vi "Anritsu VNA Read Start and Stop Frequencies.vi"(6 "Channel":i8=1 min=1 max=99 step=1, 7 "Anritsu VNA":T1, 8 "error in (no error)":errorcluster, 11 "VISA Resource Name":refnum<visa-resource-name>) -> (0 "error out":errorcluster, 2 "Start/Stop Freqs, MHz":cluster{"Fstart":dbl, "Fstop":dbl}, 3 "dup VISA Resource Name":refnum<visa-resource-name>)   [LabVIEW 2011]
doc: "This VI for the HP8753B Network Analyzers reads the stimulus values. Except when performing log sweeps and freq list sweeps, this VI uses the start and stop values and the number of points to calcuate the stimulus values."
uses:
  TypeDefs/Anritsu VNA Instrument Info.ctl
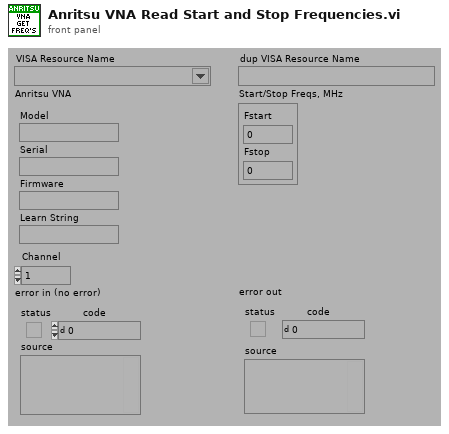
[diagram p1: front panel]
types:
  T1 = typedef "Anritsu VNA Instrument Info.ctl" = cluster{"Model":string, "Serial":string, "Firmware":string, "Learn String":string}
  T2 = typedef "Anritsu VNA Sweep Type.ctl" = enum32{"Linear Sweep", "Frequency Sweep", "Power Sweep", "CW Time Sweep", "Discrete Fill", "Time Domain", "Logarithmic Sweep", "Segmented Sweep (Frequency)", "Segmented Sweep (Index)", "MFGC"}
  T3 = typedef "Anritsu VNA Model.ctl" = enum16{"Not Supported", "37XXXX", "MS20XXX", "MS462XX", "MS464XX"}
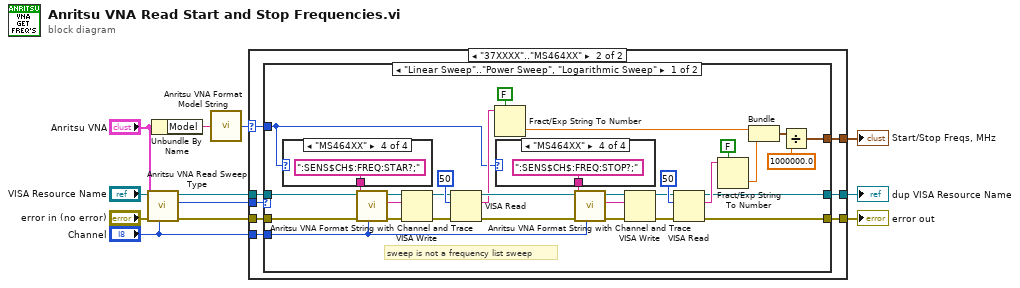
[diagram p0: block diagram]
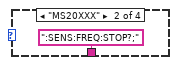
[diagram p4: hidden frame]
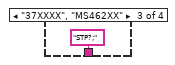
[diagram p5: hidden frame]
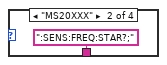
[diagram p7: hidden frame]
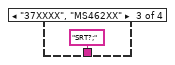
[diagram p8: hidden frame]
diagram:
  n1 = call "Anritsu VNA Read Sweep Type.vi"("Channel"="Channel", "Anritsu VNA"="Anritsu VNA", "error in (no error)"="error in (no error)", "VISA Resource Name"="VISA Resource Name") -> ("error out"=w7:errorcluster, "Sweep Type"=w10:T2, "dup VISA Resource Name"=w8:refnum<visa-resource-name>)  [unwired: 5 out]
  n2 = Unbundle By Name("Anritsu VNA") -> ("Model"=w3:string)
  n3 = call "Anritsu VNA Format Model String.vi"("Model"=w3) -> ("Model"=w2:T3)
  n4 = case shown="\"37XXXX\"..\"MS464XX\"" w2 {
    selector: w2 -> [_ w16]
    tunnel: [w13 w22] -> w12
    tunnel: w10 -> [_ w21]
    tunnel: w8 -> [w14 w20]
    tunnel: w7 -> [w13 w19]
    tunnel: [_ w18] -> w6
    tunnel: [w14 w17] -> w5
    tunnel: "Channel" -> [_ w15]
    frame "Not Supported" {
    }
    frame "37XXXX".."MS464XX" {
      n5 = case shown="\"Linear Sweep\"..\"Power Sweep\", \"Logarithmic Sweep\"" w21 {
        tunnel: w20 -> [w36 w57]
        tunnel: w19 -> [w35 w56]
        tunnel: [w43 w56] -> w22
        tunnel: [w28 _] -> w18
        tunnel: [w30 w57] -> w17
        tunnel: w16 -> [w29 _]
        tunnel: w15 -> [w23 _]
        frame "Linear Sweep".."Power Sweep", "Logarithmic Sweep" {
          # "sweep is not a frequency list sweep"
          n6 = case shown="\"MS464XX\"" w29 {
            tunnel: [_ ":SENS:FREQ:STAR?;" "SRT?;" ":SENS$CH$:FREQ:STAR?;"] -> w27
            frame "Not Supported" {
            }
            frame "MS20XXX" {
            }
            frame "37XXXX", "MS462XX" {
            }
            frame "MS464XX" {
            }
          }
          n7 = call "Anritsu VNA Format String with Channel and Trace.vi"("Channel"=w23, "String"=w27) -> ("String Out"=w26:string)  [unwired: 1 in, 6 out]
          n8 = VISA Write(VISA resource name=w36, write buffer=w26, error in (no error)=w35) -> (VISA resource name out=w39:refnum<visa-resource-name>, error out=w49:errorcluster)  [unwired: 1 out]
          n9 = VISA Read(VISA resource name=w39, byte count=u32 50, error in (no error)=w49) -> (VISA resource name out=w47:refnum<visa-resource-name>, read buffer=w45:string, error out=w46:errorcluster)  [unwired: 1 out]
          n10 = Fract/Exp String To Number(use system decimal point (T)=FALSE, string=w45) -> (number=w33:dbl)  [unwired: 3 out]
          n11 = case shown="\"MS464XX\"" w29 {
            tunnel: [_ ":SENS:FREQ:STOP?;" "STP?;" ":SENS$CH$:FREQ:STOP?;"] -> w25
            frame "Not Supported" {
            }
            frame "MS20XXX" {
            }
            frame "37XXXX", "MS462XX" {
            }
            frame "MS464XX" {
            }
          }
          n12 = call "Anritsu VNA Format String with Channel and Trace.vi"("Channel"=w23, "String"=w25) -> ("String Out"=w24:string)  [unwired: 1 in, 6 out]
          n13 = VISA Write(VISA resource name=w47, write buffer=w24, error in (no error)=w46) -> (VISA resource name out=w40:refnum<visa-resource-name>, error out=w48:errorcluster)  [unwired: 1 out]
          n14 = VISA Read(VISA resource name=w40, byte count=u32 50, error in (no error)=w48) -> (VISA resource name out=w30:refnum<visa-resource-name>, read buffer=w44:string, error out=w43:errorcluster)  [unwired: 1 out]
          n15 = Fract/Exp String To Number(use system decimal point (T)=FALSE, string=w44) -> (number=w32:dbl)  [unwired: 3 out]
          n16 = Bundle(w33, w32) -> (w31:cluster{dbl, dbl})  [unwired: 1 out]
          n17 = Divide(x=w31, y=1000000.0) -> (x/y=w28:cluster{dbl, dbl})
        }
        frame "CW Time Sweep".."Time Domain", "Segmented Sweep (Frequency)".."MFGC" {
        }
      }
    }
  }
  "dup VISA Resource Name" <- w5
  "error out" <- w12
  "Start/Stop Freqs, MHz" <- w6
